vi "Test Helper Loop Broadcast Running State.vi"(8 "error in (no error)":errorcluster, 11 "Helper Loop Test In":refnum<class "Helper Loop Test.lvclass">) -> (0 "error out":errorcluster, 3 "Helper Loop Test Out":refnum<class "Helper Loop Test.lvclass">)   [LabVIEW 2020, in "Helper Loop Test.lvclass"]
uses:
  Helper Loop Test.lvclass
  C:/Program Files (x86)/National Instruments/LabVIEW 2020/vi.lib/Asteme/LUnit/Test Case.lvclass
  Mock Process/Mock Process.lvclass
  C:/Users/anton/Documents/GitHub/Triarc-Framework/source/Framework/Process/Process.lvclass
  Framework/Process/Process.lvclass/Process.ctl
  <vilib>/Asteme/LUnit/Test Case.lvclass/Test Case.ctl
  <vilib>/Asteme/LUnit/LUnit Assertion Result.lvclass/LUnit Assertion Result.ctl
  Framework/Broadcast Event Helpers/Execution timer.vi
  Framework/Process/Private/SubVIs/Wait for finish.vi
  Framework/Process/Protected/Messaging/Enqueue Message.vi
  Framework/Process/Private/SubVIs/Set Lifecycle State.vi
  Framework/Process/Public/Lifecycle/Get Lifecycle State.vi
  <vilib>/Asteme/LUnit/Palette/Pass.vi
  <vilib>/Asteme/LUnit/Palette/Fail.vi
  <vilib>/Asteme/LUnit/Variant to string.vi
  <vilib>/Asteme/LUnit/Set Assertion Type.vi
  <vilib>/Utility/error.llb/Clear Errors.vi
  <vilib>/Asteme/LUnit/Add test result.vi
  <vilib>/Asteme/LUnit/LUnit Write Passed.vi
  <vilib>/Asteme/LUnit/LUnit Get Test Case.vi
  <vilib>/Asteme/LUnit/Assertion Result/LUnit Get Test Name.vi
  <vilib>/Asteme/LUnit/LUnit Write Message.vi
  <vilib>/Asteme/LUnit/LUnit Write Description.vi
  <vilib>/Asteme/LUnit/LUnit Write Assertion Type.vi
  <vilib>/Asteme/LUnit/Read Test Case Name.vi
  Framework/Broadcast Event Helpers/Dequeue Broadcast Message.vi
  <vilib>/Utility/error.llb/Error Cluster From Error Code.vi
  <vilib>/Utility/Data Type/Get Type Information.vi
  <vilib>/Utility/LVClass/Get LV Class Name.vi
  <vilib>/Asteme/LUnit/LUnit Assertion Result.lvclass
  Framework/Process/Process.lvclass
  <vilib>/Asteme/LUnit/Test Case.lvclass
  Framework/Broadcast Event Helpers/Broadcast Event Helpers.lvlib
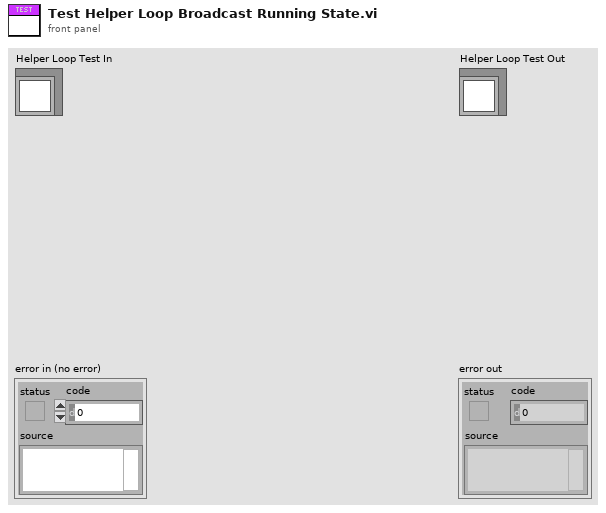
[diagram p1: front panel]
types:
  T1 = cluster{"Message":string, "Message Data":variant}
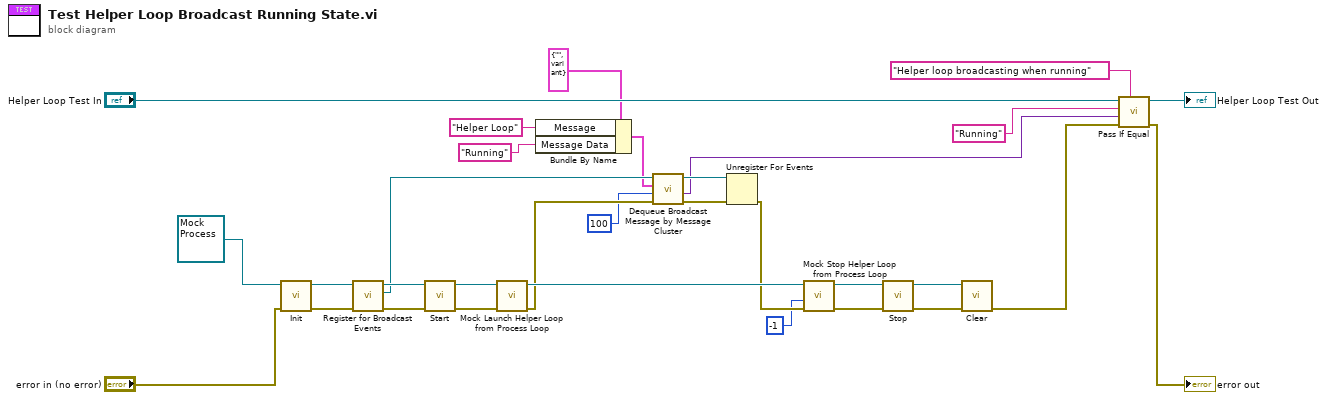
[diagram p0: block diagram]
diagram:
  n1 = call-dynamic "Init.vi"("error in (no error)"="error in (no error)", "Mock Process In"=refnum<class "Mock Process.lvclass"> refnum) -> ("error out"=w29:errorcluster, "Mock Process Out"=w30:refnum<class "Mock Process.lvclass">)  [unwired: 8 in]
  n2 = call "Register for Broadcast Events.vi"("error in (no error)"=w29, "Process In"=w30) -> ("error out"=w27:errorcluster, "Event Registration Refnum Out"=w14:refnum<event-registration>, "Process Out"=w28:refnum<class "Mock Process.lvclass">)  [unwired: 7 in]
  n3 = call "Start.vi"("error in (no error)"=w27, "Process In"=w28) -> ("error out"=w25:errorcluster, "Process Out"=w26:refnum<class "Mock Process.lvclass">)  [unwired: 7 in, 1 out]
  n4 = call "Mock Launch Helper Loop from Process Loop.vi"("error in (no error)"=w25, "Mock Process in"=w26) -> ("error out"=w12:errorcluster, "Mock Process out"=w24:refnum<class "Mock Process.lvclass">)  [unwired: 8 in]
  n5 = Bundle By Name(cluster=T1 {"Message"="", "Message Data"=variant} ("Message"), "Message"="Helper Loop" ("y"), "Message Data"="Running" ("Description")) -> (w3:T1)
  n6 = call "Dequeue Broadcast Message by Message Cluster.vi"("error in (no error)"=w12, "Timeout (-1)"=100, "Message"=w3, "Event Registration Refnum"=w14) -> ("error out"=w8:errorcluster, "Message Data"=w6:variant, "Event Registration Refnum Out"=w7:refnum<event-registration>)  [unwired: 3 in, 2 out]
  n7 = Unregister For Events(event registration refnum=w7, error in=w8) -> (error out=w11:errorcluster)
  n8 = call "Mock Stop Helper Loop from Process Loop.vi"("error in (no error)"=w11, "timeout in ms (-1)"=-1, "Mock Process in"=w24) -> ("error out"=w22:errorcluster, "Mock Process out"=w23:refnum<class "Mock Process.lvclass">)  [unwired: 6 in, 1 out]
  n9 = call "Stop.vi"("error in (no error)"=w22, "Process In"=w23) -> ("error out"=w21:errorcluster, "Process Out"=w9:refnum<class "Mock Process.lvclass">)  [unwired: 7 in, 1 out]
  n10 = call-dynamic "Clear.vi"("error in (no error)"=w21, "Mock Process In"=w9) -> ("error out"=w20:errorcluster)  [unwired: 9 in]
  n11 = call <vilib>:"Pass If Equal.vi"("Description"="Helper loop broadcasting when running", "error in (no error)"=w20, "Actual"=w6, "Expected"="Running" ("Description"), "Test Case In"="Helper Loop Test In") -> ("error out"=→"error out":errorcluster, "Test Case Out"=→"Helper Loop Test Out":refnum<class "Helper Loop Test.lvclass">)  [unwired: 5 in]
